vi "Read Scope Bitmap.vi"(8 "error in (no error)":errorcluster, 9 "Timeout (10000 ms)":u32=10000, 11 "VISA resource name":refnum<visa-resource-name>) -> (0 "error out":errorcluster, 2 "scope":picture, 3 "VISA resource name out":refnum<visa-resource-name>)   [LabVIEW 2015, in "ZhiYuan ZDS Series for TCP.lvlib"]
uses:
  ZhiYuan ZDS Series for TCP.lvlib
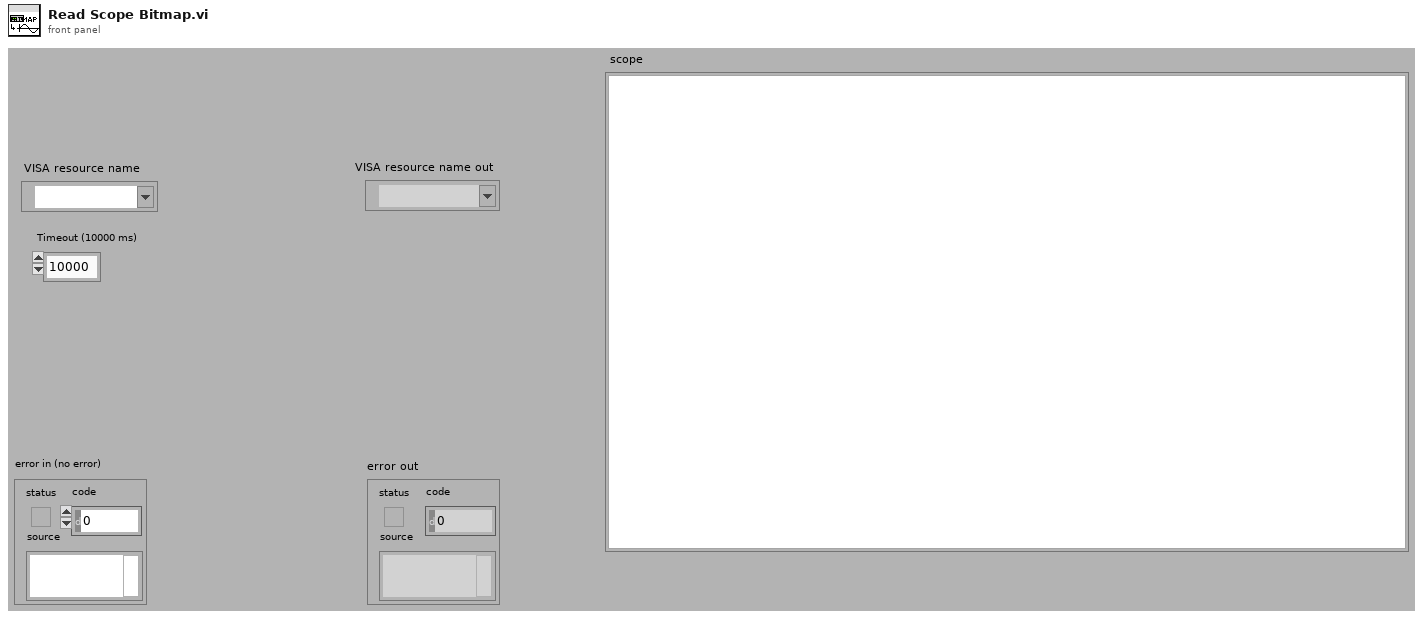
[diagram p1: front panel]
types:
  T1 = typedef "imagedata.ctl" = cluster{"image type":i32, "image depth":i32, "image":u8[], "mask":u8[], "colors":u32[], "Rectangle":cluster{"left":i16, "top":i16, "right":i16, "bottom":i16}}
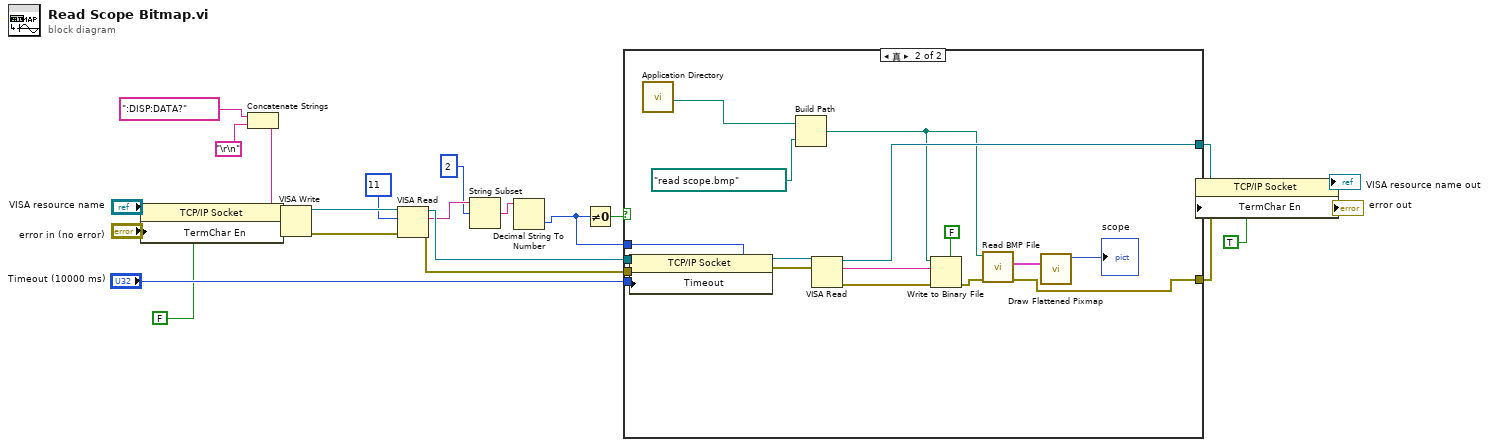
[diagram p0: block diagram]
diagram:
  n1 = property class="TCP/IP Socket"(reference="VISA resource name", error in="error in (no error)", "TermChar En"=FALSE ("Message Based Settings:Termination Character Enable")) -> (reference out=w8:refnum<visa-resource-name>, error out=w6:errorcluster)
  n2 = Concatenate Strings(":DISP:DATA?", "\r\n") -> (w21:string)
  n3 = VISA Write(VISA resource name=w8, write buffer=w21, error in (no error)=w6) -> (VISA resource name out=w24:refnum<visa-resource-name>, error out=w23:errorcluster)  [unwired: 1 out]
  n4 = VISA Read(VISA resource name=w24, byte count=u32 11, error in (no error)=w23) -> (VISA resource name out=w18:refnum<visa-resource-name>, read buffer=w14:string, error out=w17:errorcluster)  [unwired: 1 out]
  n5 = String Subset(string=w14, offset (0)=2) -> (substring=w12:string)  [unwired: 1 in]
  n6 = Decimal String To Number(string=w12) -> (number=w11:i32)  [unwired: 2 in, 1 out]
  n7 = Not Equal To 0?(x=w11) -> (x != 0?=w19:bool)
  n8 = case shown="真" w19 {
    tunnel: w18 -> [w26 w43]
    tunnel: w17 -> [w25 w42]
    tunnel: "Timeout (10000 ms)" -> [_ w39]
    tunnel: w11 -> [_ w38]
    tunnel: [w25 w35] -> w2
    tunnel: [w26 w34] -> w3
    frame False {
    }
    frame True {
      n9 = property class="TCP/IP Socket"(reference=w43, error in=w42, "Timeout"=w39) -> (reference out=w41:refnum<visa-resource-name>, error out=w40:errorcluster)
      n10 = call <vilib>:"Application Directory.vi"() -> ("Application Directory"=w27:path)
      n11 = Build Path(base path=w27, name or relative path=path "read scope.bmp" ("file (use dialog)")) -> (appended path=w28:path)
      n12 = VISA Read(VISA resource name=w41, byte count=w38, error in (no error)=w40) -> (VISA resource name out=w34:refnum<visa-resource-name>, read buffer=w33:string, error out=w32:errorcluster)  [unwired: 1 out]
      n13 = Write to Binary File(file (use dialog)=w28, data=w33, error in=w32, 5:FALSE ("prepend array or string size? (T)")) -> (error out=w31:errorcluster)  [unwired: 2 in, 2 out]
      n14 = call <vilib>:"Read BMP File.vi"("error in (no error)"=w31, "path to BMP file"=w28) -> ("error out"=w35:errorcluster, "image data"=w37:T1)  [unwired: 7 in, 1 out]
      n15 = call <vilib>:"Draw Flattened Pixmap.vi"("image data"=w37) -> ("new picture"=→"scope":picture)  [unwired: 8 in]
    }
  }
  n16 = property class="TCP/IP Socket"(reference=w3, error in=w2, "TermChar En"=TRUE ("Message Based Settings:Termination Character Enable")) -> (reference out=→"VISA resource name out":refnum<visa-resource-name>, error out=→"error out":errorcluster)
